vi "Complex FFT.vi"(9 "FFT size":i32=-1, 10 "shift?":bool, 11 "X":cdb[](array[numeric])) -> (0 "error":i32, 3 "FFT {X}":cdb[](array[numeric]))   [LabVIEW 2010, in "NI_AALPro.lvlib"]
doc: "Computes the fast Fourier transform (FFT) of the input sequence <B>X</B>. Wire data to the <B>X</B> input to determine the polymorphic instance to use or manually select the instance."
uses:
  NI_AALPro.lvlib
  lvanlys.dll
panel:
  # "Complex FFT"
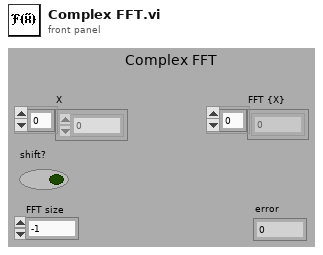
[diagram p1: front panel]
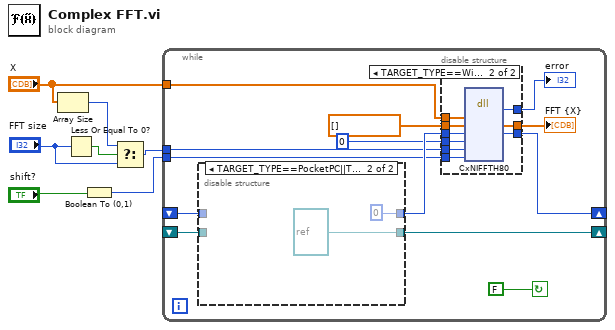
[diagram p0: block diagram]
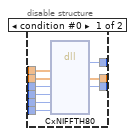
[diagram p2: hidden frame]
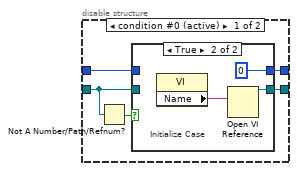
[diagram p3: hidden frame]
diagram:
  n1 = Array Size(array="X") -> (size(s)=w6:i32)
  n2 = Less Or Equal To 0?(x="FFT size") -> (x <= 0?=w7:bool)
  n3 = Boolean To (0,1)(Boolean="shift?") -> (0, 1=w1:i16)
  n4 = Select(t=w6, s=w7, f="FFT size") -> (s? t:f=w3:i32)
  n5 = while {
    shift-left: _ -> [w17]
    shift-right: [w18] -> _
    tunnel: "X" -> [w20]
    shift-right: [w14] -> _
    shift-left: _ -> [w15]
    tunnel: w3 -> [w11]
    tunnel: w1 -> [w13]
    stop <- FALSE continue-if-true
    n6 = disable-structure shown="TARGET_TYPE==PocketPC||TARGET_TYPE==PalmOS||TARGET_TYPE==FPGA||TARGET_TYPE==Embedded" {
      disable-tunnel: w15 -> [w41 _]
      disable-tunnel: [w42 refnum<vi> refnum ("VI Refnum")] -> w14
      disable-tunnel: w17 -> [w40 _]
      disable-tunnel: [w39 0 ("t")] -> w16
      frame condition #0 (active) {
        n7 = Not A Number/Path/Refnum?(number/path/refnum=w41) -> (NaN/Path/Refnum?=w43:bool)
        n8 = case shown="True" w43 {
          tunnel: [w45 w47] -> w42
          tunnel: w41 -> [w45 _]
          tunnel: w40 -> [w44 _]
          tunnel: [w44 0 ("error")] -> w39
          frame False {
          }
          frame True {
            # "Initialize Case"
            n9 = property class="VI"() -> ("Name"=w46:string)  [unwired: 2 in, 2 out]
            n10 = Open VI Reference(vi path=w46) -> (vi reference=w47:refnum<vi>)  [unwired: 5 in, 1 out]
          }
        }
      }
      frame condition #1 {
      }
    }
    n11 = disable-structure shown="TARGET_TYPE==Windows||TARGET_TYPE==Mac||TARGET_TYPE==Unix" {
      disable-tunnel: w20 -> [w29 w38]
      disable-tunnel: [w28 w37] -> w9
      disable-tunnel: [w27 w36] -> w18
      disable-tunnel: w16 -> [w26 w35]
      disable-tunnel: w13 -> [w25 w34]
      disable-tunnel: [w24 w33] -> w12
      disable-tunnel: w11 -> [w23 w32]
      disable-tunnel: 0 ("org") -> [w22 w31]
      disable-tunnel: cdb[] [] ("FFT {X}") -> [w21 w30]
      frame condition #0 {
        n12 = dll-call lib="C:/Program Files/National Instruments/LabVIEW 2010/resource/lvanlys.dll" fn="CxNIFFTH80"("X"=w29, w21, "tbl"=w26, "org"=w22, "fftSize"=w23, "shift"=w25) -> (w24:i32, w28:cdb[], "tbl"=w27:i32)  [unwired: 7 in, 2 out]
      }
      frame condition #1 (active) {
        n13 = dll-call lib="C:/Program Files/National Instruments/LabVIEW 2010/resource/lvanlys.dll" fn="CxNIFFTH80"("xH"=w38, "yH"=w30, "tbl"=w35, "org"=w31, "fftSize"=w32, "shift"=w34) -> ("return type"=w33:i32, "yH"=w37:cdb[], "tbl"=w36:i64)  [unwired: 7 in, 2 out]
      }
    }
    "FFT {X}" <- w9
    "error" <- w12
  }
